vi "Lab_FinalUI_NaimaAhmedNup.vi"() -> ()   [LabVIEW 2020]
panel:
  in  "VISA resource name":refnum<visa-resource-name>
  in  "Table Control":string[][](table)
  out "Humidity Waveform":dbl(graph)
  out "Temparature Waveform":dbl(graph)
  out "Humidity":dbl(knob) scale=0.0..10.0
  out "Temparature":dbl(slide) scale=0.0..100.0
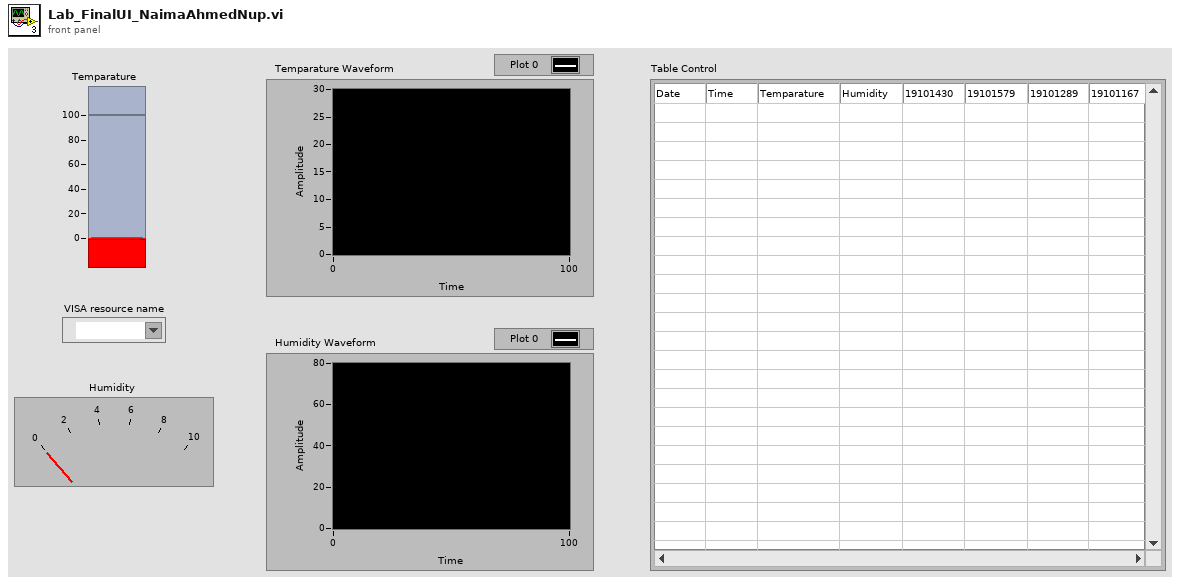
[diagram p1: front panel]
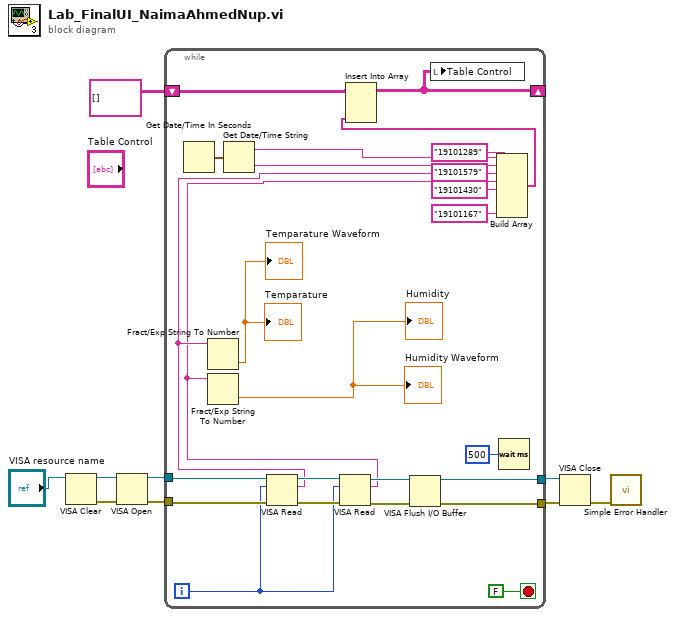
[diagram p0: block diagram]
diagram:
  n1 = VISA Clear(VISA resource name="VISA resource name") -> (VISA resource name out=w8:refnum<visa-resource-name>, error out=w9:errorcluster)  [unwired: 1 in]
  n2 = VISA Open(error in (no error)=w9, VISA resource name=w8) -> (VISA resource name=w6:refnum<visa-resource-name>, error out=w5:errorcluster)  [unwired: 3 in]
  n3 = while {
    tunnel: w6 -> [w30]
    tunnel: w5 -> [w29]
    tunnel: [w28] -> w4
    tunnel: [w27] -> w3
    shift-right: [w21] -> _
    shift-left: string[][] [] -> [w22]
    i -> [w26]
    stop <- FALSE stop-if-true
    n4 = Get Date/Time In Seconds() -> (seconds since 1Jan1904=w20:timestamp)
    n5 = Get Date/Time String(seconds (now)=w20) -> (date string=w19:string, time string=w18:string)  [unwired: 2 in]
    n6 = VISA Read(VISA resource name=w30, byte count=w26, error in (no error)=w29) -> (VISA resource name out=w33:refnum<visa-resource-name>, read buffer=w16:string, error out=w34:errorcluster)  [unwired: 1 out]
    n7 = Fract/Exp String To Number(string=w16) -> (number=→"Temparature" →"Temparature Waveform":dbl)  [unwired: 3 in, 1 out]
    n8 = VISA Read(VISA resource name=w33, byte count=w26, error in (no error)=w34) -> (VISA resource name out=w31:refnum<visa-resource-name>, read buffer=w15:string, error out=w32:errorcluster)  [unwired: 1 out]
    n9 = Fract/Exp String To Number(string=w15) -> (number=→"Humidity" →"Humidity Waveform":dbl)  [unwired: 3 in, 1 out]
    n10 = VISA Flush I/O Buffer(VISA resource name=w31, error in (no error)=w32) -> (VISA resource name out=w28:refnum<visa-resource-name>, error out=w27:errorcluster)  [unwired: 1 in]
    n11 = Build Array(w19, w18, w16, w15, "19101430" ("element"), "19101579" ("element"), "19101289" ("element"), "19101167" ("element")) -> (w17:string[])
    n12 = Insert Into Array(array=w22, new element=w17) -> (w21:string[][])  [unwired: 2 in]
    n13 = local write "Table Control"(w21) -> ()
    n14 = Wait (ms)(milliseconds to wait=u32 500) -> ()  [unwired: 1 out]
  }
  n15 = VISA Close(VISA resource name=w4, error in (no error)=w3) -> (error out=w7:errorcluster)
  n16 = call <vilib>:"Simple Error Handler.vi"("error in (no error)"=w7) -> ()  [unwired: 4 in, 5 out]
